vi "Read Power.vi"(8 "error in":errorcluster, 11 "Modbus instance in":refnum<class "Modbus API.lvclass">) -> (0 "error out":errorcluster, 2 "Power Read":dbl, 3 "Modbus instance out":refnum<class "Modbus API.lvclass">)   [LabVIEW 2025, in "Hanmatek HM310T.lvlib"]
uses:
  <vilib>/NI/Modbus Library/API/Modbus API.lvclass
  <instrlib>/Hanmatek HM310T/Hanmatek HM310T.lvlib
  e1d78ae1-c481-44ed-b7f3-8e7e0b2ea88c.vi
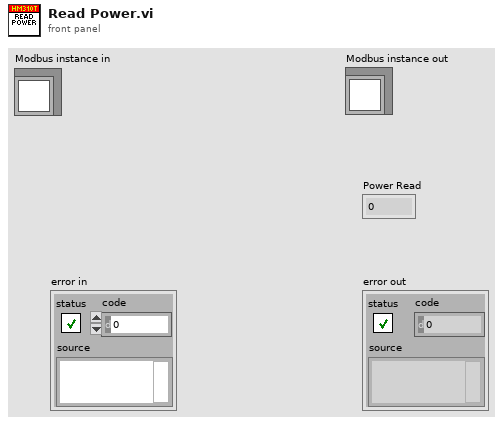
[diagram p1: front panel]
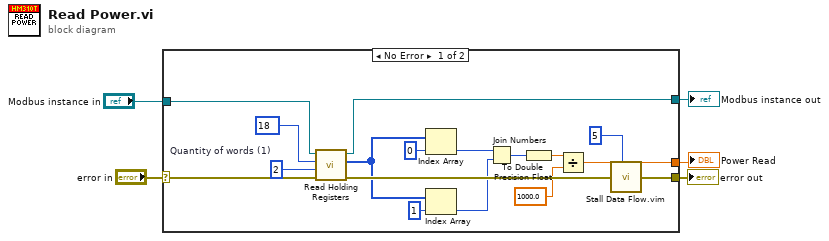
[diagram p0: block diagram]
diagram:
  n1 = case shown="No Error" "error in" {
    selector: "error in" -> [w21 w24]
    tunnel: [w7 w24] -> w4
    tunnel: [w19 w23] -> w2
    tunnel: [w15 _] -> w3
    tunnel: "Modbus instance in" -> [w8 w23]
    frame No Error {
      w14 = u16 2  # Quantity of words (1)
      n2 = call-dynamic "Read Holding Registers.vi"("error in"=w21, "number of inputs"=w14, "starting address"=u16 18 ("Quantity of words (1)"), "Modbus instance in"=w8) -> ("error out"=w20:errorcluster, "register values"=w12:u16[], "Modbus instance out"=w19:refnum<class "Modbus API.lvclass">)  [unwired: 5 in]
      n3 = Index Array(array=w12, index=0) -> (element=w10:u16)
      n4 = Index Array(array=w12, index=1) -> (element=w9:u16)
      n5 = Join Numbers(hi=w10, lo=w9) -> ((hi.lo)=w11:u32)
      n6 = To Double Precision Float(number=w11) -> (double precision float=w16:dbl)
      n7 = Divide(x=w16, y=1000.0) -> (x/y=w15:dbl)
      n8 = call "Stall Data Flow.vim"("value in"=w20, "milliseconds to wait"=u32 5) -> ("value out"=w7:errorcluster)  [unwired: 1 out]
    }
    frame Error {
    }
  }
  "error out" <- w4
  "Power Read" <- w3
  "Modbus instance out" <- w2
